vi "Actor Core.vi"(8 "error in":errorcluster, 11 "Chat Window Model in":refnum<class "Chat Window Model.lvclass">) -> (0 "error out":errorcluster, 3 "Actor out":refnum<class "Actor.lvclass">)   [LabVIEW 2020, in "Chat Window Model.lvlib" / "Chat Window Model.lvclass"]
doc: "(<B>Filename</B>: Actor Framework.lvlib:Actor.lvclass:Actor Core.vi)\n\nReceives messages to the actor, reacts to them, and initiates any error handling that may shut the actor down.\n\nDescendant classes may override this VI to append parallel tasks for the actor to complete while it handles messages. Overrides use the Call Parent Method node."
uses:
  Chat Window Model.lvclass
  C:/Program Files/National Instruments/LabVIEW 2020/vi.lib/ActorFramework/Actor/Actor.lvclass
  <vilib>/ActorFramework/Actor/Actor.lvclass
  Chat Window Interface/Chat Window Interface/Chat Window Interface.lvclass
  C:/Users/huipeng8/Desktop/Video 12 - LabVIEW Maps/Chat Window UI Controller/Chat Window UI Controller/Chat Window UI Controller.lvclass
  Chat Window Model.lvclass/Chat Window Model.ctl
  Chat Window UI Controller/Chat Window UI Controller/Chat Window UI Controller.lvclass/Chat Window UI Controller.ctl
  Chat Window UI Controller/Chat Window UI Controller/Chat Window UI Controller.lvclass
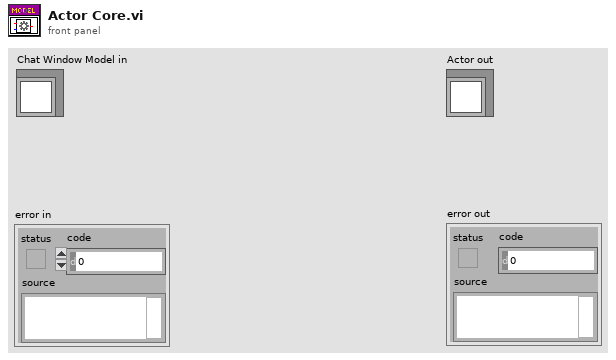
[diagram p1: front panel]
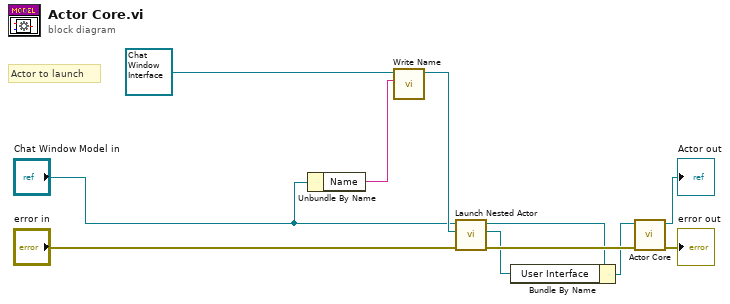
[diagram p0: block diagram]
diagram:
  # "Actor to launch"
  n1 = Unbundle By Name("Chat Window Model in") -> ("Name"=w2:string)
  n2 = call "Write Name.vi"("Name"=w2, "Chat Window UI Controller in"=refnum<class "Chat Window Interface.lvclass"> refnum ("Chat Window Interface.lvlib:Chat Window Interface.lvclass")) -> ("Chat Window UI Controller out"=w4:refnum<class "Chat Window Interface.lvclass">)  [unwired: 8 in, 1 out]
  n3 = call <vilib>:"Launch Nested Actor.vi"("error in (no error)"="error in", "Nested Actor"=w4, "Caller Actor in"="Chat Window Model in") -> ("error out"=w8:errorcluster, "Nested Actor's Enqueuer"=w5:refnum<class "Message Enqueuer.lvclass">, "Caller Actor out"=w6:refnum<class "Chat Window Model.lvclass">)  [unwired: 6 in]
  n4 = Bundle By Name(cluster=w6, "User Interface"=w5) -> (w7:refnum<class "Chat Window Model.lvclass">)
  n5 = call-parent "Actor Core.vi"("error in"=w8, "Actor in"=w7) -> ("error out"=→"error out":errorcluster, "Actor out"=→"Actor out":refnum<class "Actor.lvclass">)  [unwired: 8 in]
